vi "Read Section.vi"   [LabVIEW 2024, in "Generic Config Handling.lvlib"]
doc: "This vi reads the cluster from a section in the config file. \n\nIf section name is not wired then the default is to use the name of the cluster.\n\nEach element of the cluster becomes a key, therefore it must be named, and they should be unique and not include any special characters (spaces are allowed and are replaced by_)\n\nYou cannot nest clusters and only simple datatypes are allowed. 1D and 2D arrays are allowed. They are stored as a single element with columns delimited by semicolons and rows delimited by commas. 1D arrays are stored as a single row (ie. comma delimited). \n\nEnums are stored as U32s.\n\nThe cluster wired to Section is used as the default values for the keys if they are not found. If any key is missing, missing keys is true and a list of missing keys is provided."
uses:
  Generic Config Handling.lvlib
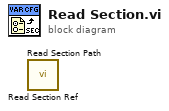
[diagram p0: block diagram]
diagram:
  n1 = call "Read Section Ref.vi"() -> ()  [unwired: 7 in, 5 out]
  n2 = call "Read Section Path.vi"() -> ()  [unwired: 7 in, 5 out]
